vi "Game of Life.vi"() -> ()   [LabVIEW 2014]
doc: "A simple environment creator with an exploratory, food-hunting robot."
panel:
  out "World (after)":i8[][](graph)
  out "World (beginning)":i8[][](graph)
  out "Step":i32
  out "Sensor Array":i8[][](array[numeric])
  out "World (current) Matrix":i8[][](array[numeric])
  out "Sensor Reading Chart":i8[][](graph)
  in  "Food per Level":i32
  in  "Level":i32
  in  "Cycle Delay":u32(slide) step=25 scale=50.0..2000.0
  out "V_Heading":i8
  out "Sense Heading":i8
  out "Y:":i8
  out "X:":i8
  out "Energy":i8(slide) scale=0.0..30.0
  in  "Emergency Stop":bool
  out "Robot running \nwhen BLINKING":bool
  in  "Control Panels":enum32{"Initial World Data", "World Graph"}(tab)
  out "World (initial)":i8[][](graph)
  out "World (current)":i8[][](graph)
  # "Difficulty"
  # "Robot Position"
  # "Headings"
  # "Vcode\n  6 7 8\n  5 0 1\n  4 3 2"
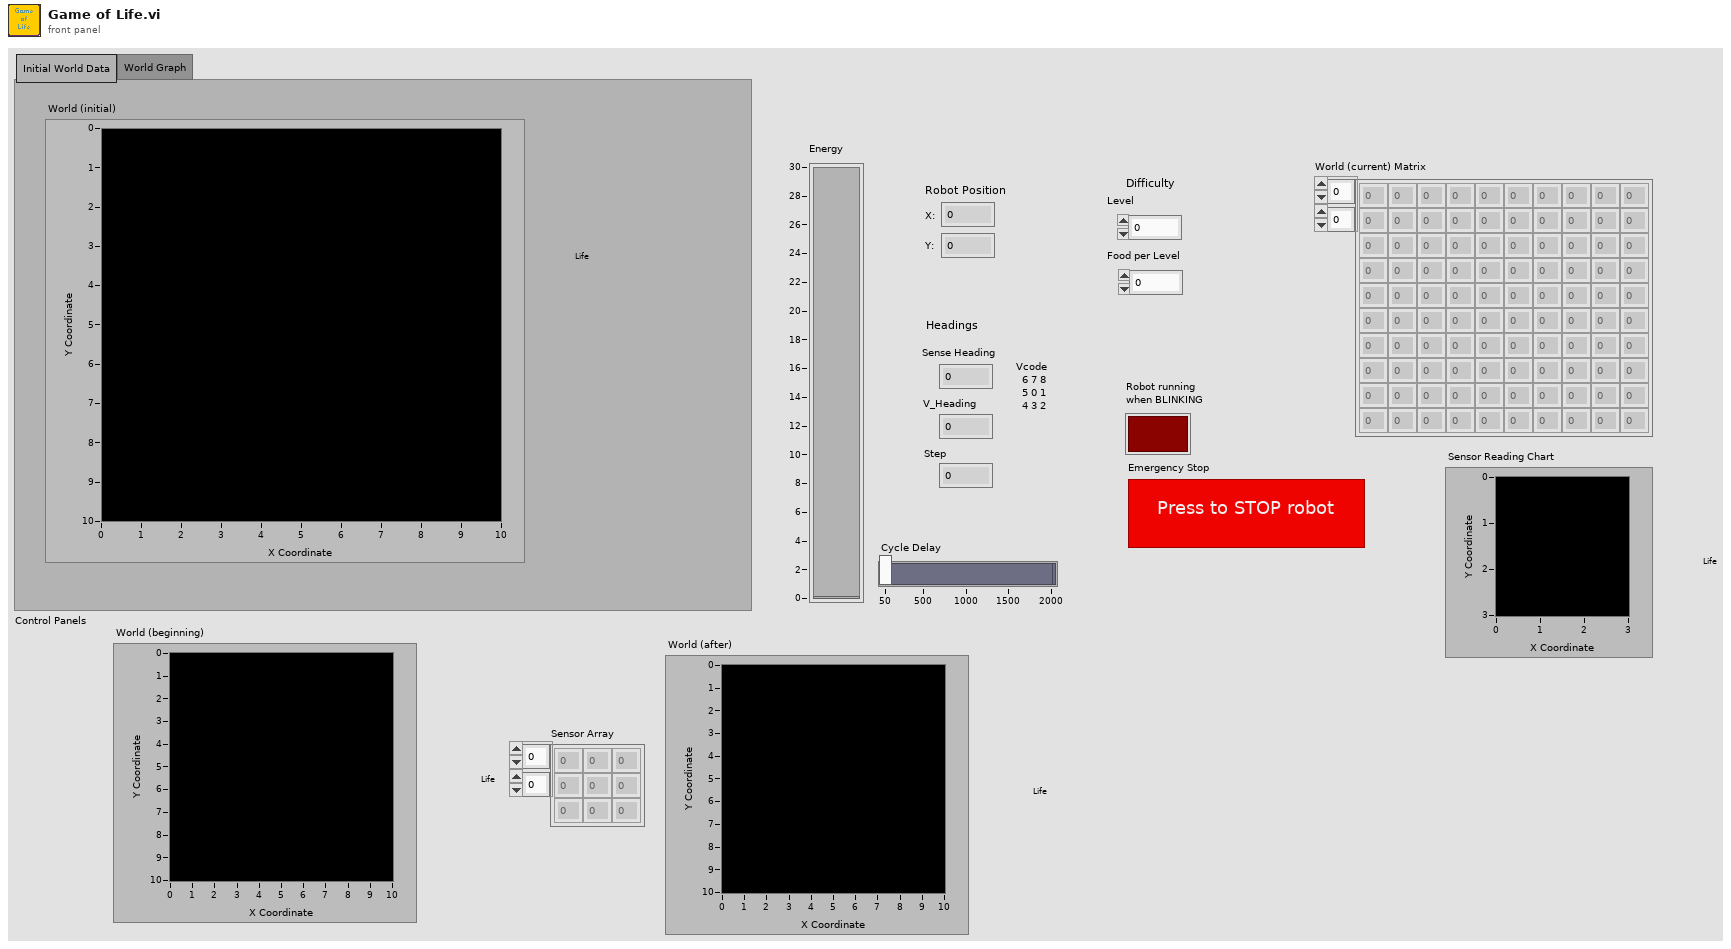
[diagram p1: front panel]
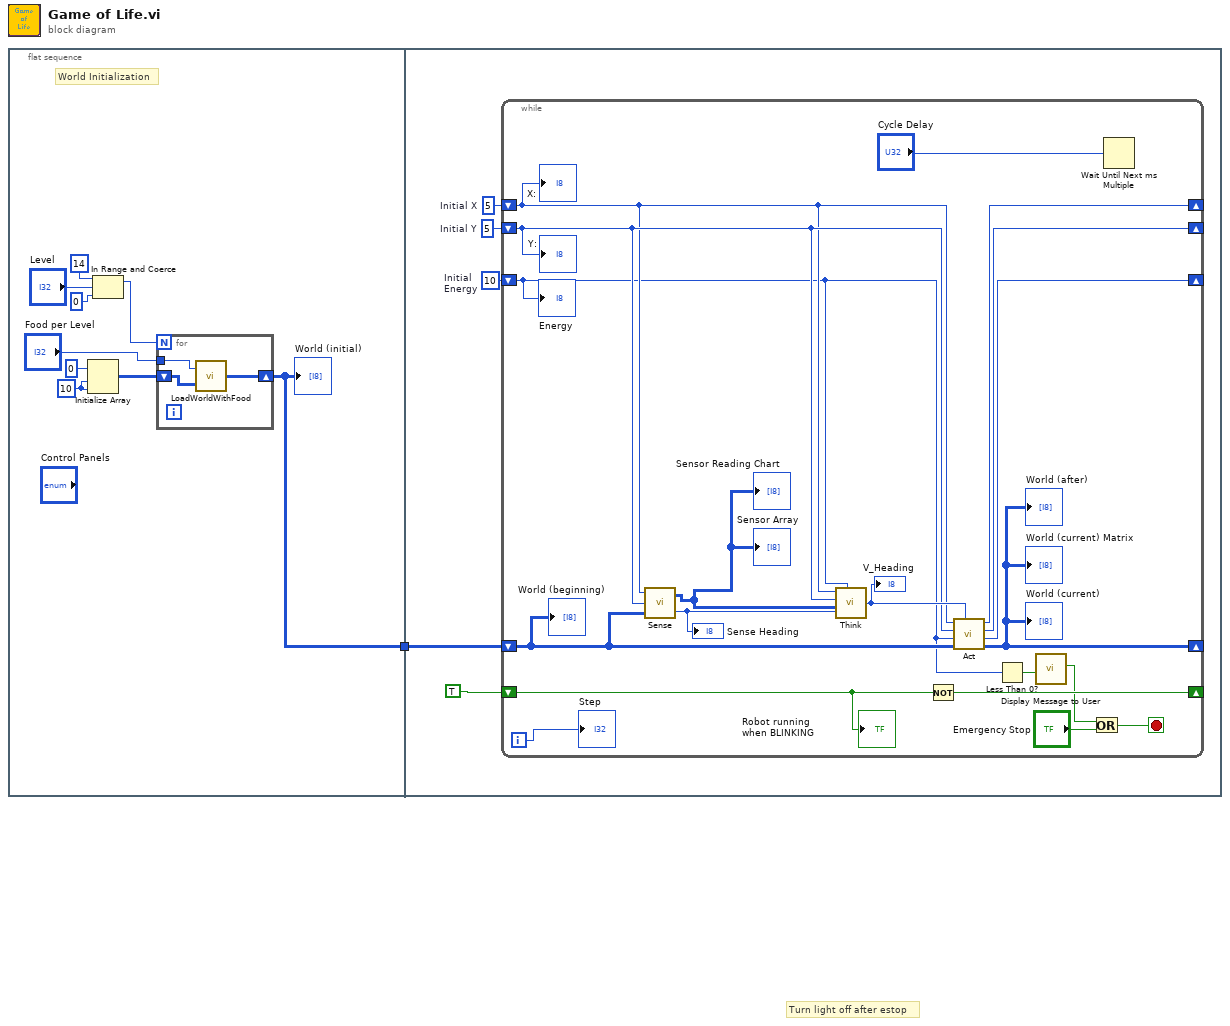
[diagram p0: block diagram]
diagram:
  # "Turn light off after estop"
  n1 = flat-sequence {
    tunnel: [w2] -> w1
    tunnel: w1 -> [w17]
    frame #0 {
      w9 = 10
      # "World Initialization"
      n2 = Initialize Array ("Initialize Array (Initialize World)")(i8 0, w9, w9) -> (w4:i8[][])
      n3 = In Range and Coerce(upper limit=14, x="Level", lower limit=0) -> (coerced(x)=w5:i32)  [unwired: 1 out]
      n4 = for {
        N: w5 -> [_]
        shift-right: [w11] -> w2
        shift-left: w4 -> [w12]
        tunnel: "Food per Level" -> [w13]
        n5 = call "LoadWorldWithFood.vi"("Input Array"=w12, "Food per Level"=w13) -> ("Output Array"=w11:i8[][])
      }
      "World (initial)" <- w2
    }
    frame #1 {
      w14 = i8 10  # Initial  Energy
      w15 = i8 5  # Initial Y
      w16 = i8 5  # Initial X
      n6 = while {
        shift-right: [w36] -> _
        shift-left: TRUE -> [w37]
        shift-right: [w24] -> _
        shift-left: w17 -> [w23]
        shift-right: [w28] -> _
        shift-left: w16 -> [w21]
        shift-right: [w27] -> _
        shift-left: w15 -> [w22]
        shift-right: [w26] -> _
        shift-left: w14 -> [w20]
        i -> [w25]
        stop <- w32 stop-if-true
        n7 = call "Sense.vi"("World"=w23, "Y"=w22, "X"=w21) -> ("Heading"=w30:i8, "Sensor Array"=w19:i8[][])
        "Sense Heading" <- w30
        "Sensor Reading Chart" <- w19
        "Sensor Array" <- w19
        n8 = call "Think.vi"("X"=w21, "Y"=w22, "Sensor View"=w19, "Sense Heading"=w30, "E"=w20) -> ("V Heading"=w29:i8)
        "V_Heading" <- w29
        n9 = Not(x=w37) -> (.not. x?=w36:bool)
        n10 = call "Act.vi"("V"=w29, "InWorld"=w23, "E_in"=w20, "Y_in"=w22, "X_in"=w21) -> ("Outworld"=w24:i8[][], "E_out"=w26:i8, "Y_out"=w27:i8, "X_out"=w28:i8)
        "World (current)" <- w24
        "World (current) Matrix" <- w24
        "World (after)" <- w24
        n11 = Less Than 0?(x=w20) -> (x < 0?=w34:bool)
        n12 = call "Display Message to User"("Enable"=w34) -> ("Damn, that's sad."=w31:bool)  [unwired: 9 in, 1 out]
        n13 = Or(x=w31, y="Emergency Stop") -> (x .or. y?=w32:bool)
        n14 = Wait Until Next ms Multiple(millisecond multiple="Cycle Delay") -> ()  [unwired: 1 out]
        "Energy" <- w20
        "Robot running \nwhen BLINKING" <- w37
        "X:" <- w21
        "Y:" <- w22
        "Step" <- w25
        "World (beginning)" <- w23
      }
    }
  }
